vi "APP_Training.vi"(8 "error in":errorcluster) -> (0 "error out":errorcluster, 2 "Data":waveform(dbl), 3 "OK?":bool)   [LabVIEW 2015, in "Application 2.lvlib"]
uses:
  Application 2.lvlib
  Data Def/App_Simulator Data Method.ctl
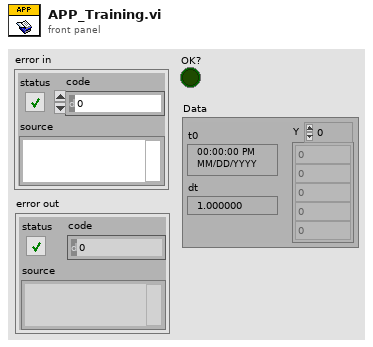
[diagram p1: front panel]
types:
  T1 = typedef "Application 2.lvlib/App_Simulator Data Method.ctl" = enum16{"Get", "Put"}
  T2 = typedef "Application 2.lvlib/App_Main Data.ctl" = cluster{"VI Refnum":refnum<vi>, "Subpanel":refnum<vi>, "Connection ID":refnum<k5>, "Meta data":T3[], "Main Queue":T5, "User Data":T6}
  T3 = typedef "stm_MetaElement.ctl" = cluster{"Name":T4}
  T4 = typedef "stm_MetaDataElement.ctl" = string
  T5 = typedef "Application 2.lvlib/App_Main Queue.ctl" = cluster{"Main Loop Queue":refnum<queue>}
  T6 = typedef "User Data.ctl" = cluster{"Name":string, "Email":string, "Phone Number":string, "User Picture":u32[][], "Last Login Time":timestamp}
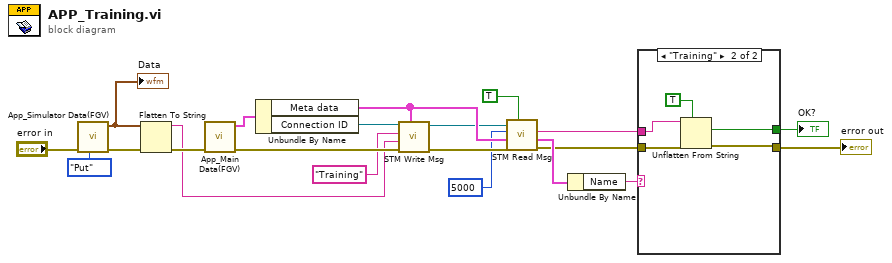
[diagram p0: block diagram]
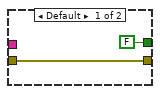
[diagram p2: hidden frame]
diagram:
  n1 = call "App_Simulator Data(FGV).vi"("Simulator Data Method(Get)"=App_Simulator_Data_Method."Put" ("Simulator Data Method"), "error in"="error in") -> ("error out"=w15:errorcluster, "Data"=w14:waveform(dbl))  [unwired: 8 in]
  "Data" <- w14
  n2 = Flatten To String(anything=w14, error in (no error)=w15) -> (data string=w13:string, error out=w16:errorcluster)  [unwired: 2 in, 1 out]
  n3 = call "App_Main Data(FGV).vi"("error in"=w16) -> ("error out"=w20:errorcluster, "Main Data Out"=w21:T2)  [unwired: 9 in]
  n4 = Unbundle By Name(w21) -> ("Meta data"=w10:T3[], "Connection ID"=w19:refnum<k5>)
  n5 = call "STM Write Msg.vi"("Meta data"=w10, "error in (no error)"=w20, "Data"=w13, "Name"="Training", "connection ID"=w19) -> ("error out"=w11:errorcluster, "connection ID out"=w9:refnum<k5>)  [unwired: 5 in]
  n6 = call "STM Read Msg.vi"("Ignore Timeout Error"=TRUE, "error in"=w11, "Meta data"=w10, "timeout ms (25000)"=5000, "connection ID"=w9) -> ("error out"=w5:errorcluster, "Meta element"=w6:T3, "data string"=w3:string)  [unwired: 1 in, 3 out]
  n7 = Unbundle By Name(w6) -> ("Name"=w4:T4)
  n8 = case shown="\"Training\"" w4 {
    tunnel: w5 -> [w23 w28]
    tunnel: w3 -> [_ w27]
    tunnel: [w23 w25] -> w1
    tunnel: [FALSE w24] -> w2
    frame Default {
    }
    frame "Training" {
      n9 = Unflatten From String(type=TRUE, binary string=w27, error in (no error)=w28) -> (value=w24:bool, error out=w25:errorcluster)  [unwired: 2 in, 1 out]
    }
  }
  "error out" <- w1
  "OK?" <- w2
